vi "obtain queues.vi"(11 "initialise? (F)":bool) -> (3 "queues":T1)   [LabVIEW 2018]
uses:
  type defs/Queues.ctl
  supporting VIs/polymorphic VIs/enqueue for message handler.vi
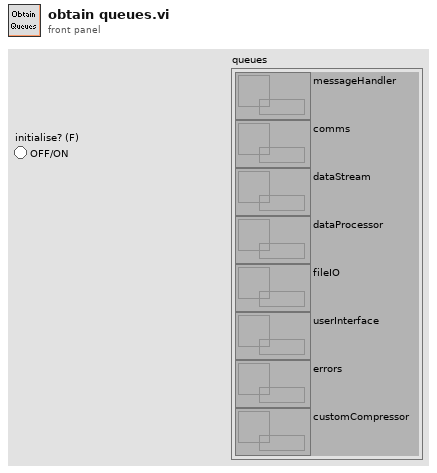
[diagram p1: front panel]
types:
  T1 = typedef "Queues.ctl" = cluster{"messageHandler":refnum<queue>, "comms":refnum<queue>, "dataStream":refnum<queue>, "dataProcessor":refnum<queue>, "fileIO":refnum<queue>, "userInterface":refnum<queue>, "errors":refnum<queue>, "customCompressor":refnum<queue>}
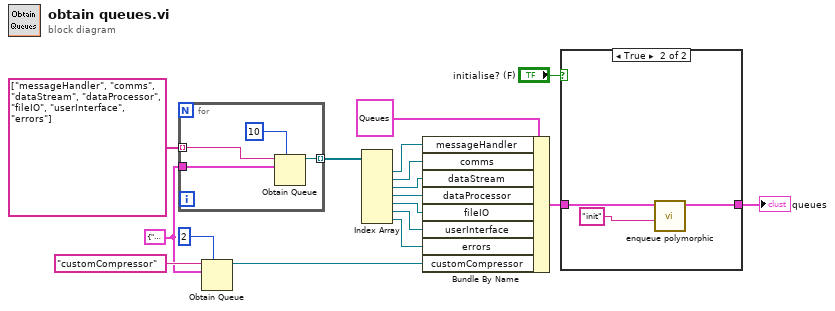
[diagram p0: block diagram]
diagram:
  w5 = cluster{"message":string, "data":variant} {"message"="", "data"=variant}
  n1 = for {
    tunnel: string[] ["messageHandler", "comms", "dataStream", "dataProcessor", "fileIO", "userInterface", "errors"] ("name (unnamed)") -> [w20] mode=indexing
    tunnel: [w19] -> w16 mode=indexing
    tunnel: w5 -> [w18]
    n2 = Obtain Queue(max queue size (-1, unlimited)=10, name (unnamed)=w20, element data type=w18) -> (queue out=w19:refnum<queue>)  [unwired: 2 in, 2 out]
  }
  n3 = Obtain Queue(max queue size (-1, unlimited)=2, name (unnamed)="customCompressor", element data type=w5) -> (queue out=w6:refnum<queue>)  [unwired: 2 in, 2 out]
  n4 = Index Array(array=w16) -> (element #1=w14:refnum<queue>, element #2=w13:refnum<queue>, element #3=w12:refnum<queue>, element #4=w11:refnum<queue>, element #5=w10:refnum<queue>, element #6=w9:refnum<queue>, element #7=w8:refnum<queue>)  [unwired: 7 in]
  n5 = Bundle By Name(cluster=T1 {"messageHandler"=refnum, "comms"=refnum, "dataStream"=refnum, "dataProcessor"=refnum, "fileIO"=refnum, "userInterface"=refnum, "errors"=refnum, "customCompressor"=refnum} ("Queues"), "messageHandler"=w14, "comms"=w13, "dataStream"=w12, "dataProcessor"=w11, "fileIO"=w10, "userInterface"=w9, "errors"=w8, "customCompressor"=w6) -> (w3:T1)
  n6 = case shown="True" "initialise? (F)" {
    tunnel: w3 -> [w22 w24]
    tunnel: [w22 w23] -> w2
    frame False {
    }
    frame True {
      n7 = call-poly "enqueue polymorphic.vi"("message"="init", "Queues"=w24) -> ("Queues out"=w23:T1)  [unwired: 9 in]
    }
  }
  "queues" <- w2
